vi "csm_lumikki_instron_startRamp_poller.vi"   [LabVIEW 2009]
types:
  T1 = cluster{"Name":string, "Type":i32, "SI Full Scale":dbl, "Full Scale":dbl, "Units String":string, "Display Format":string, "Gauge Length":dbl}[][]
  T2 = cluster{"Device ID":i32, "Device Name":string, "Device Type":i32}[]
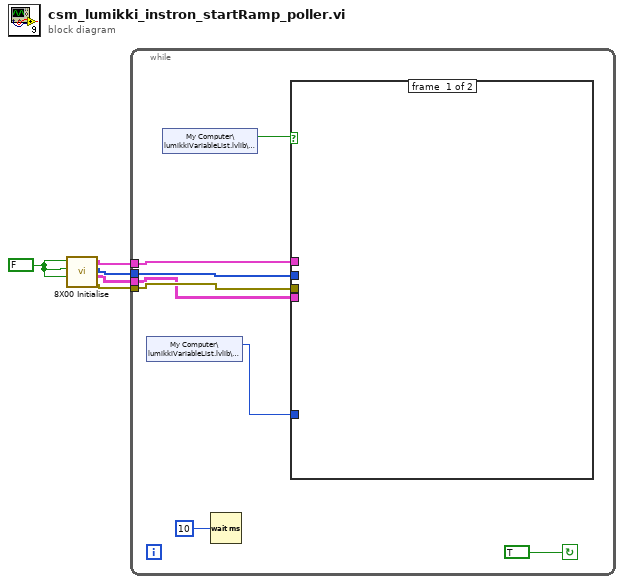
[diagram p0: block diagram]
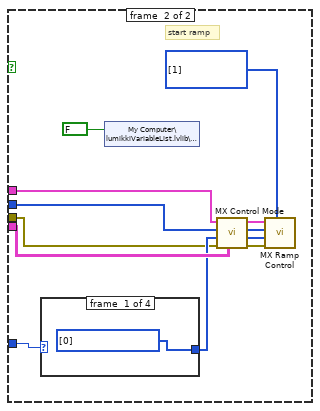
[diagram p2: hidden frame]
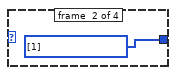
[diagram p3: hidden frame]
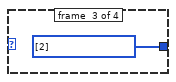
[diagram p4: hidden frame]
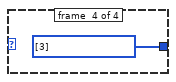
[diagram p5: hidden frame]
diagram:
  w1 = FALSE ("Create Console? (T)")
  n1 = call "8X00 Initialise.vi"("Reset?"=w1, "Create DVM? (T)"=w1, "Create Console? (T)"=w1) -> ("error out"=w3:errorcluster, "Channel Data"=w2:T1, "Axis Selector"=w4:i32[], "Axis Information"=w5:T2)  [unwired: 1 in]
  n2 = while {
    tunnel: w5 -> [w12]
    tunnel: w4 -> [w11]
    tunnel: w3 -> [w10]
    tunnel: w2 -> [w7]
    stop <- TRUE continue-if-true
    n3 = shared-variable "My Computer\\lumikkiVariableList.lvlib\\channelInt"() -> (w6:i32)  [unwired: 1 in, 1 out]
    n4 = shared-variable "My Computer\\lumikkiVariableList.lvlib\\startRamp"() -> (w9:bool)  [unwired: 1 in, 1 out]
    n5 = Wait (ms)(milliseconds to wait=u32 10) -> ()  [unwired: 1 out]
    n6 = case shown="True" w9 {
      tunnel: w12 -> [_ w14]
      tunnel: w11 -> [_ w15]
      tunnel: w10 -> [_ w16]
      tunnel: w6 -> [_ w24]
      tunnel: w7 -> [_ w22]
      frame #0 {
      }
      frame #1 {
        w25 = u16[] [1] items=["Stop", "Start or continue", "Hold", "Continue", "Return ramp to set level at fixed rate", "Reserved", "Reserved", "Start Random without demand hold", "Start Random with demand hold", "Prepare Random Start without demand hold", "Prepare Random Start with demand hold", "Unslave", "Reserved", "Reserved", "Start Sample Data Playback or Resume", "Prepare for Start of Sample Data", "Reserved", "Reserved", "Resume Playback", "Start an electromechanical frame return"] ("Ramp Control")
        # "start ramp"
        n7 = case shown="1, Default" w24 {
          tunnel: [w26 w27 w28 w29] -> w17
          frame #0 {
            w26 = u16[] [0] items=["Channel 1", "Channel 2", "Channel 3", "Channel 4"] ("Choose channel to apply\nthe setpoint")
          }
          frame #1 {
            w27 = u16[] [1] items=["Channel 1", "Channel 2", "Channel 3", "Channel 4"] ("Choose channel to apply\nthe setpoint")
          }
          frame #2 {
            w28 = u16[] [2] items=["Channel 1", "Channel 2", "Channel 3", "Channel 4"] ("Choose channel to apply\nthe setpoint")
          }
          frame #3 {
            w29 = u16[] [3] items=["Channel 1", "Channel 2", "Channel 3", "Channel 4"] ("Choose channel to apply\nthe setpoint")
          }
        }
        n8 = shared-variable "My Computer\\lumikkiVariableList.lvlib\\startRamp"(FALSE ("startRamp")) -> ()  [unwired: 1 in, 1 out]
        n9 = call "MX Control Mode.vi"("Channel Data"=w22, "error in (no error)"=w16, "Control Modes"=w17, "Axis Selector"=w15, "Axis Information"=w14) -> ("error out"=w21:errorcluster, "Control Modes out"=w20:u16[], "Axis Selector out"=w19:i32[], "Axis Information out"=w18:T2)  [unwired: 1 in]
        n10 = call "MX Ramp Control.vi"("Ramp Control"=w25, "error in (no error)"=w21, "Channels In"=w20, "Axis Selector In"=w19, "Axis Information In"=w18) -> ()  [unwired: 2 in, 4 out]
      }
    }
  }
